vi "Get Point Value Map Reference.vi"(8 "error in (no error)":errorcluster) -> (0 "error out":errorcluster, 3 "Map Out":T1)   [LabVIEW 2021, in "DigitalAudioGenerationProcess.lvlib"]
uses:
  DigitalAudioGenerationProcess.lvlib
  <vilib>/addons/PointValueMap/PointValueMap.lvlib
  <vilib>/addons/PointValueMap/controls/PointMap.ctl
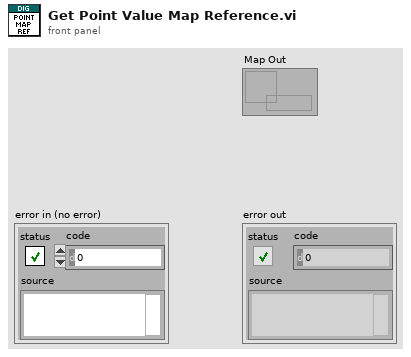
[diagram p1: front panel]
types:
  T1 = typedef "PointValueMap.lvlib/PointMap.ctl" = refnum<data-value>
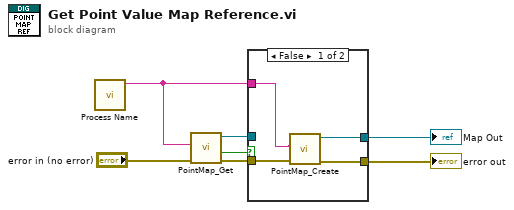
[diagram p0: block diagram]
diagram:
  n1 = call "Process Name.vi"() -> ("process name"=w1:string)  [unwired: 11 in]
  n2 = call <vilib>:"PointMap_Get.vi"("error in (no error)"="error in (no error)", "Name"=w1) -> ("error out"=w6:errorcluster, "Found?"=w7:bool, "Map Out"=w5:T1)  [unwired: 7 in]
  n3 = case shown="False" w7 {
    tunnel: w6 -> [w11 w12]
    tunnel: [w10 w12] -> w3
    tunnel: w5 -> [_ w13]
    tunnel: [w9 w13] -> w2
    tunnel: w1 -> [w8 _]
    frame False {
      n4 = call <vilib>:"PointMap_Create.vi"("error in (no error)"=w11, "Name"=w8) -> ("error out"=w10:errorcluster, "Map Out"=w9:T1)  [unwired: 8 in]
    }
    frame True {
    }
  }
  "error out" <- w3
  "Map Out" <- w2
